vi "SubTest_UpdateData.vi"() -> ()   [LabVIEW 2014, in "TableLogger_CSV_Actor.lvlib" / "TableLogger_CSV_Actor.lvclass"]
uses:
  TableLogger_CSV_Actor.lvclass
  TableLogger_Actor/TableLoggerConfig.ctl
  TableLogger_Actor/TableLoggerTypes.ctl
  TableLogger_Actor/TableLoggerBackupConfig.ctl
  TableLogger_Actor/TableLogger_Actor.lvlib
panel:
  in  "error in (no error)":errorcluster
  out "error out":errorcluster
  # "This example to check CSV update on Tablelogger"
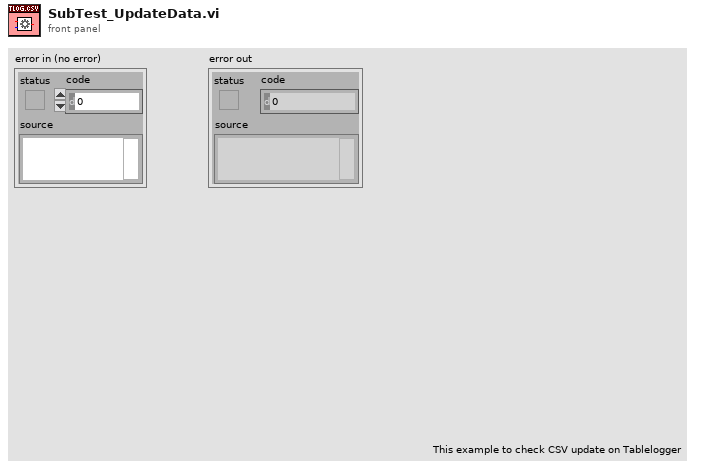
[diagram p1: front panel]
types:
  T1 = cluster{"Numeric Data":i32, "Float Data":dbl, "String Data":string, "Enum Data":enum16{"Enum Item 1", "Enum Item 2"}, "Array Data":i32[], "Array Data 2":i32[]}
  T2 = cluster{"Numeric Data":i32, "Float Data":dbl, "String Data":string, "Enum Data":enum16{"Enum Item 1", "Enum Item 2"}, "Array Data":i32[], "Array Data 2":i32[]}[]
  T3 = typedef "TableLogger_Actor.lvlib/TableLoggerConfig.ctl" = cluster{"TableLogger":T4, "DB File Path":path, "DB Backup Config":T5}
  T4 = typedef "TableLogger_Actor.lvlib/TableLoggerTypes.ctl" = enum16{"CSV Logger", "SQLite Logger"}
  T5 = typedef "TableLogger_Actor.lvlib/TableLoggerBackupConfig.ctl" = cluster{"Directory":path, "UTC Time Format":bool, "On Launch":bool, "Interval (Hours)":dbl, "Size Multiples (Bytes)":i32}
  T6 = cluster{"Numeric Data":i32, "Float Data":dbl, "String Data":string, "Enum Data":enum16{"Enum Item 1", "Enum Item 2"}, "Array Data":i32[]}
  T7 = cluster{"Test Start Timestamp":timestamp, "Test End Timestamp":timestamp, "Test Jig Location":string, "Location Time Offset":string, "Test Jig ID":string, "Test Jig Fluid":enum16{"Liquid", "Gas"}, "Test Jig Flow":enum16{"Low", "High"}, "Control Board SN":string, "Site Number":i32, "Operator ID":string, "Operation Number":string, "DUT Serial Number":string, "DUT Product Number":string, "DUT Flow Range":i32, "DUT FW Revision":string, "DUT TP1 Offset":dbl, "DUT TP2 Offset":dbl, "DUT Cut Off1":dbl, "DUT Cut Off2":dbl, "PreCal Flow Meas":cluster{"FC Flow Set":dbl, "FM Flow Measure":dbl, "UUT Data":dbl}[], "PostCal Flow Meas":cluster{"FC Flow Set":dbl, "FM Flow Measure":dbl, "UUT Data":dbl}[], "DUT_Coeff":dbl[], "DUT_Flow_Error":dbl[], "Calibration Result":enum16{"Pass", "Fail"}}
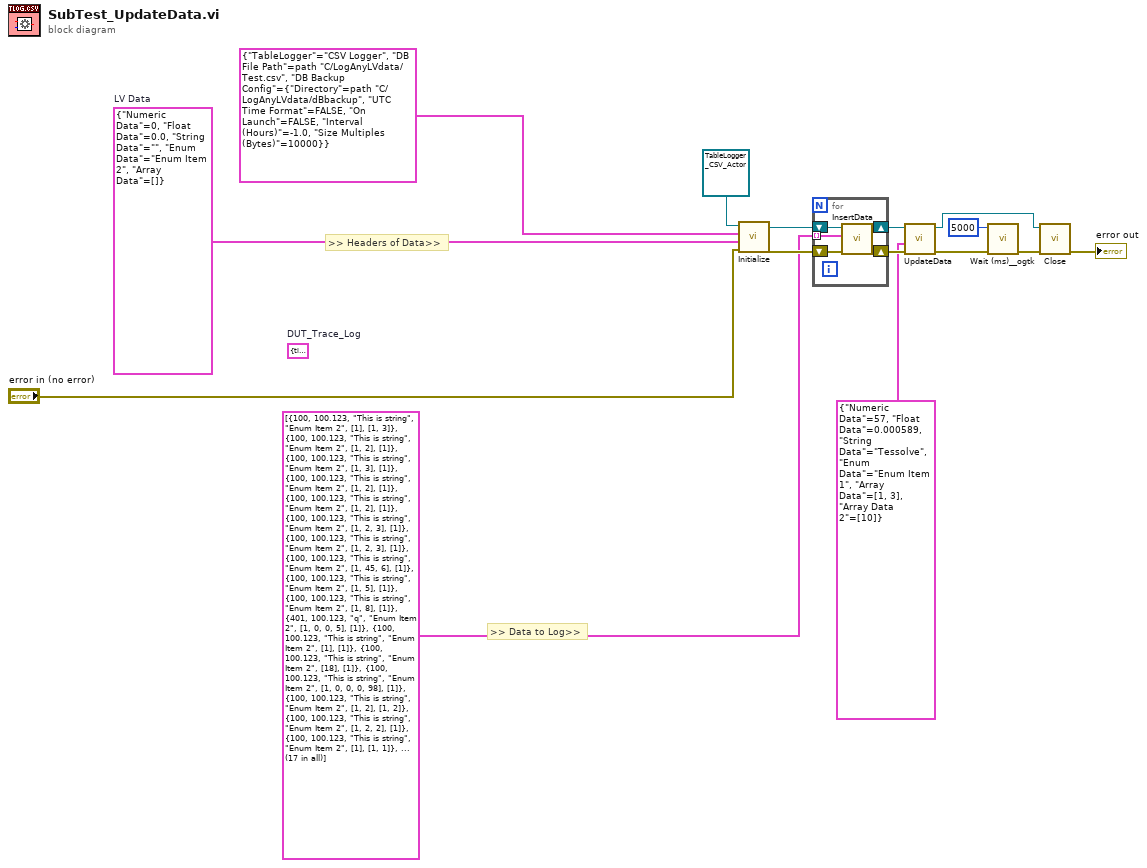
[diagram p0: block diagram]
diagram:
  w9 = T6 {"Numeric Data"=0, "Float Data"=0.0, "String Data"="", "Enum Data"=enum."Enum Item 2", "Array Data"=[]}  # LV Data
  (unwired) T7 {"Test Start Timestamp"=timestamp(0 s since 1904-01-01), "Test End Timestamp"=timestamp(0 s since 1904-01-01), "Test Jig Location"="asdf", "Location Time Offset"="wer", "Test Jig ID"="xcv", "Test Jig Fluid"=enum."Gas", "Test Jig Flow"=enum."High", "Control Board SN"="fgh", "Site Number"=23, "Operator ID"="op", "Operation Number"="op", "DUT Serial Number"="dt", "DUT Product Number"="dt", "DUT Flow Range"=23, "DUT FW Revision"="asdf", "DUT TP1 Offset"=24.0, "DUT TP2 Offset"=546.0, "DUT Cut Off1"=34.0, "DUT Cut Off2"=453.0, "PreCal Flow Meas"=[{"FC Flow Set"=1.0, "FM Flow Measure"=0.0, "UUT Data"=0.0}, {"FC Flow Set"=2.0, "FM Flow Measure"=0.0, "UUT Data"=0.0}, {"FC Flow Set"=3.0, "FM Flow Measure"=0.0, "UUT Data"=0.0}], "PostCal Flow Meas"=[{"FC Flow Set"=1.0, "FM Flow Measure"=0.0, "UUT Data"=0.0}, {"FC Flow Set"=2.0, "FM Flow Measure"=0.0, "UUT Data"=0.0}], "DUT_Coeff"=[1.0, 2.0], "DUT_Flow_Error"=[1.0, 2.0], "Calibration Result"=enum."Fail"}  # DUT_Trace_Log
  # ">> Headers of Data>>"
  # ">> Data to Log>>"
  n1 = call-dynamic "Initialize.vi"("error in (no error)"="error in (no error)", "Data Cluster (for Headers)"=w9, "TableLogger Config"=T3 {"TableLogger"=enum."CSV Logger", "DB File Path"=path "C:/LogAnyLVdata/Test.csv", "DB Backup Config"={"Directory"=path "C:/LogAnyLVdata/dBbackup", "UTC Time Format"=FALSE, "On Launch"=FALSE, "Interval (Hours)"=-1.0, "Size Multiples (Bytes)"=10000}}, "object in"=refnum<class "TableLogger_CSV_Actor.lvclass"> refnum) -> ("error out"=w12:errorcluster, "object out"=w13:refnum<class "TableLogger_CSV_Actor.lvclass">)  [unwired: 6 in]
  n2 = for {
    shift-right: [w18] -> w3
    shift-left: w13 -> [w20]
    shift-right: [w17] -> w4
    shift-left: w12 -> [w19]
    tunnel: T2 [{"Numeric Data"=100, "Float Data"=100.123, "String Data"="This is string", "Enum Data"=enum."Enum Item 2", "Array Data"=[1], "Array Data 2"=[1, 3]}, {"Numeric Data"=100, "Float Data"=100.123, "String Data"="This is string", "Enum Data"=enum."Enum Item 2", "Array Data"=[1, 2], "Array Data 2"=[1]}, {"Numeric Data"=100, "Float Data"=100.123, "String Data"="This is string", "Enum Data"=enum."Enum Item 2", "Array Data"=[1, 3], "Array Data 2"=[1]}, {"Numeric Data"=100, "Float Data"=100.123, "String Data"="This is string", "Enum Data"=enum."Enum Item 2", "Array Data"=[1, 2], "Array Data 2"=[1]}, {"Numeric Data"=100, "Float Data"=100.123, "String Data"="This is string", "Enum Data"=enum."Enum Item 2", "Array Data"=[1, 2], "Array Data 2"=[1]}, {"Numeric Data"=100, "Float Data"=100.123, "String Data"="This is string", "Enum Data"=enum."Enum Item 2", "Array Data"=[1, 2, 3], "Array Data 2"=[1]}, {"Numeric Data"=100, "Float Data"=100.123, "String Data"="This is string", "Enum Data"=enum."Enum Item 2", "Array Data"=[1, 2, 3], "Array Data 2"=[1]}, {"Numeric Data"=100, "Float Data"=100.123, "String Data"="This is string", "Enum Data"=enum."Enum Item 2", "Array Data"=[1, 45, 6], "Array Data 2"=[1]}, {"Numeric Data"=100, "Float Data"=100.123, "String Data"="This is string", "Enum Data"=enum."Enum Item 2", "Array Data"=[1, 5], "Array Data 2"=[1]}, {"Numeric Data"=100, "Float Data"=100.123, "String Data"="This is string", "Enum Data"=enum."Enum Item 2", "Array Data"=[1, 8], "Array Data 2"=[1]}, {"Numeric Data"=401, "Float Data"=100.123, "String Data"="q", "Enum Data"=enum."Enum Item 2", "Array Data"=[1, 0, 0, 5], "Array Data 2"=[1]}, {"Numeric Data"=100, "Float Data"=100.123, "String Data"="This is string", "Enum Data"=enum."Enum Item 2", "Array Data"=[1], "Array Data 2"=[1]}, {"Numeric Data"=100, "Float Data"=100.123, "String Data"="This is string", "Enum Data"=enum."Enum Item 2", "Array Data"=[18], "Array Data 2"=[1]}, {"Numeric Data"=100, "Float Data"=100.123, "String Data"="This is string", "Enum Data"=enum."Enum Item 2", "Array Data"=[1, 0, 0, 0, 98], "Array Data 2"=[1]}, {"Numeric Data"=100, "Float Data"=100.123, "String Data"="This is string", "Enum Data"=enum."Enum Item 2", "Array Data"=[1, 2], "Array Data 2"=[1, 2]}, {"Numeric Data"=100, "Float Data"=100.123, "String Data"="This is string", "Enum Data"=enum."Enum Item 2", "Array Data"=[1, 2, 2], "Array Data 2"=[1]}, {"Numeric Data"=100, "Float Data"=100.123, "String Data"="This is string", "Enum Data"=enum."Enum Item 2", "Array Data"=[1], "Array Data 2"=[1, 1]}] -> [w16] mode=indexing
    n3 = call-dynamic "InsertData.vi"("error in (no error)"=w19, "Data Cluster"=w16, "object in"=w20) -> ("error out"=w17:errorcluster, "object out"=w18:refnum<class "TableLogger_CSV_Actor.lvclass">)  [unwired: 7 in]
  }
  n4 = call "UpdateData.vi"("error in (no error)"=w4, "Data Cluster"=T1 {"Numeric Data"=57, "Float Data"=0.000589, "String Data"="Tessolve", "Enum Data"=enum."Enum Item 1", "Array Data"=[1, 3], "Array Data 2"=[10]} ("LV Data"), "object in"=w3) -> ("error out"=w14:errorcluster, "object out"=w5:refnum<class "TableLogger_CSV_Actor.lvclass">)  [unwired: 7 in]
  n5 = call <userlib>:"Wait (ms)__ogtk.vi"("error in (no error)"=w14, "milliseconds to wait"=u32 5000) -> ("error out"=w7:errorcluster)  [unwired: 8 in, 1 out]
  n6 = call-dynamic "Close.vi"("error in (no error)"=w7, "object in"=w5) -> ("error out"=→"error out":errorcluster)  [unwired: 8 in, 1 out]
